vi "S1&S2_CHECK.vi"(8 "Message 2":string, 9 "MODE":string, 11 "task/channels in":refnum<k21>="CHECK_STS_S1") -> (3 "S1Bit_out":string)   [LabVIEW 2011]
uses:
  <vilib>/DAQmx/read.llb/DAQmx Read (Digital 1D Bool 1Chan 1Samp).vi
panel:
  out "Message":string
  out "Time out":dbl(slide) scale=0.0..40.0
  out "DIP SWITCH":bool[](array[boolean])
  # "1"
  # "2"
  # "3"
  # "4"
  # "5"
  # "6"
  # "7"
  # "8"
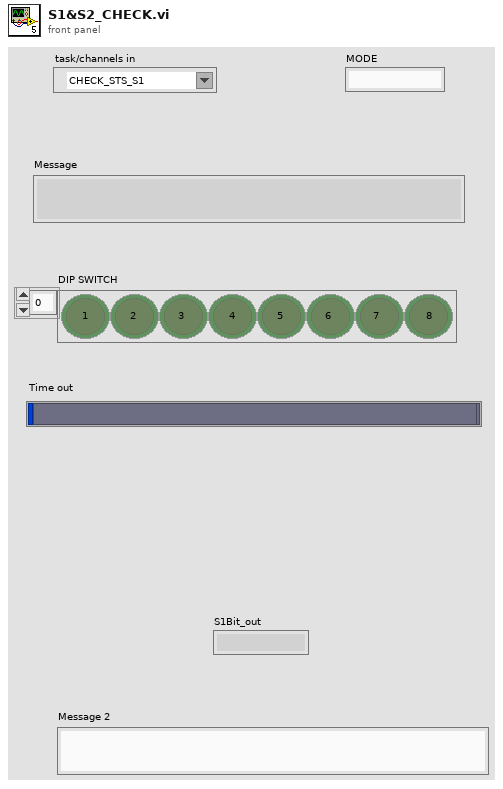
[diagram p1: front panel]
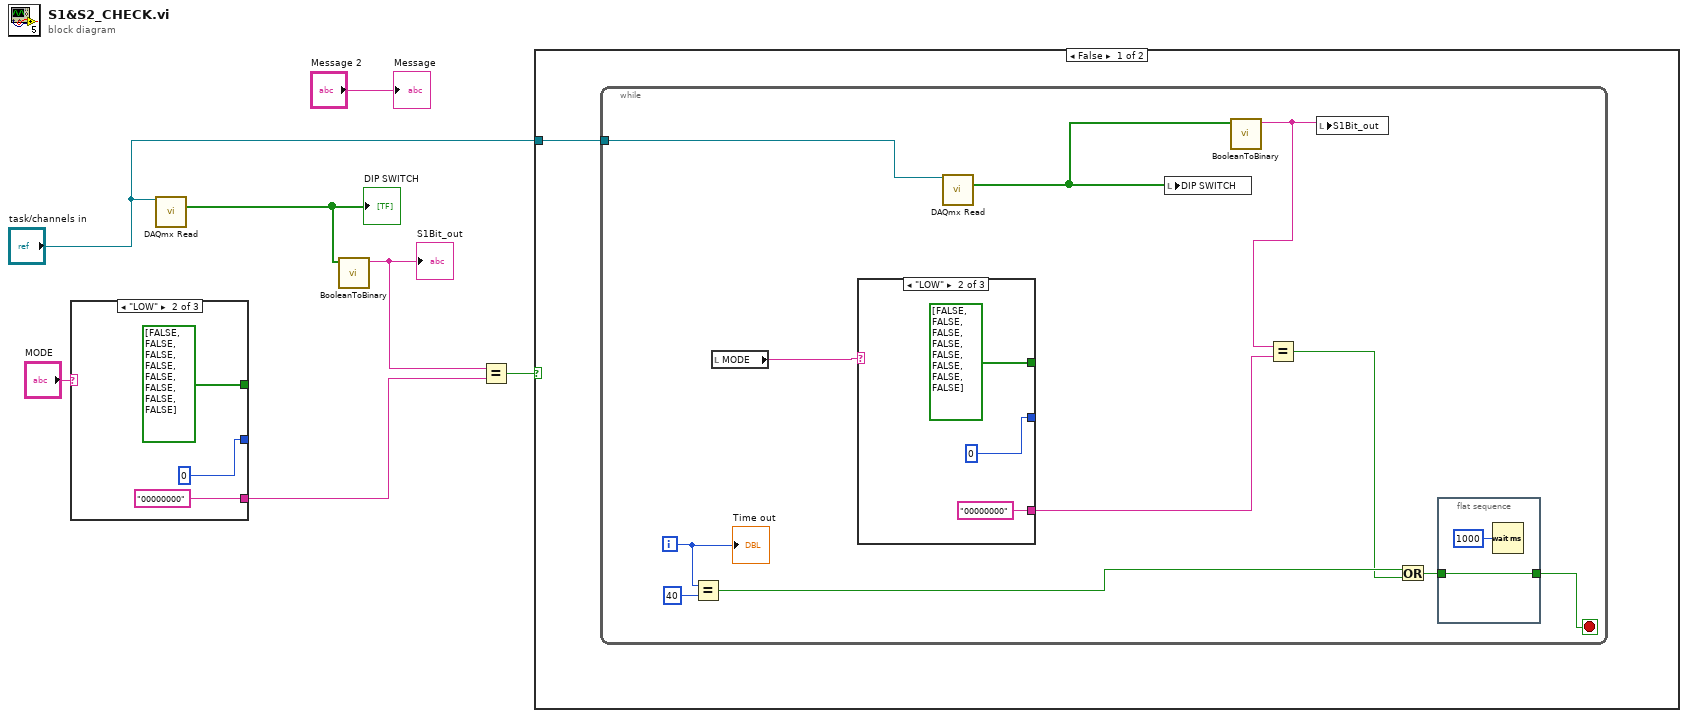
[diagram p0: block diagram]
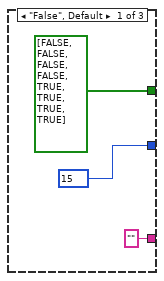
[diagram p2: hidden frame]
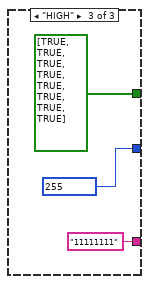
[diagram p3: hidden frame]
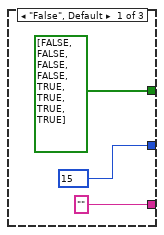
[diagram p5: hidden frame]
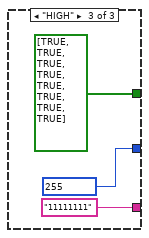
[diagram p6: hidden frame]
diagram:
  n1 = case shown="\"LOW\"" "MODE" {
    tunnel: [bool[] [FALSE, FALSE, FALSE, FALSE, TRUE, TRUE, TRUE, TRUE] ("y") bool[] [FALSE, FALSE, FALSE, FALSE, FALSE, FALSE, FALSE, FALSE] ("y") bool[] [TRUE, TRUE, TRUE, TRUE, TRUE, TRUE, TRUE, TRUE] ("y")] -> _
    tunnel: [u32 15 ("FF") u32 0 ("FF") u32 255 ("FF")] -> _
    tunnel: ["" "00000000" "11111111"] -> w1
    frame "False", Default {
    }
    frame "LOW" {
    }
    frame "HIGH" {
    }
  }
  n2 = call-poly <vilib>:"DAQmx Read.vi"("task/channels in"="task/channels in") -> ("data"=w3:bool[])  [unwired: 12 in, 2 out]
  "DIP SWITCH" <- w3
  n3 = call "BooleanToBinary.vi"("data"=w3) -> ("BinaryOut"=w2:string)  [unwired: 10 in]
  "S1Bit_out" <- w2
  n4 = Equal?(x=w2, y=w1) -> (x = y?=w7:bool)
  n5 = case shown="False" w7 {
    tunnel: "task/channels in" -> [w17 _]
    frame False {
      n6 = while {
        tunnel: w17 -> [w21]
        i -> [w28]
        stop <- w23 stop-if-true
        n7 = Equal?(x=w28, y=40) -> (x = y?=w26:bool)
        n8 = local read "MODE"() -> (w25:string)
        n9 = case shown="\"LOW\"" w25 {
          tunnel: [bool[] [FALSE, FALSE, FALSE, FALSE, TRUE, TRUE, TRUE, TRUE] ("y") bool[] [FALSE, FALSE, FALSE, FALSE, FALSE, FALSE, FALSE, FALSE] ("y") bool[] [TRUE, TRUE, TRUE, TRUE, TRUE, TRUE, TRUE, TRUE] ("y")] -> _
          tunnel: [u32 15 ("FF") u32 0 ("FF") u32 255 ("FF")] -> _
          tunnel: ["" "00000000" "11111111"] -> w18
          frame "False", Default {
          }
          frame "LOW" {
          }
          frame "HIGH" {
          }
        }
        n10 = call-poly <vilib>:"DAQmx Read.vi"("task/channels in"=w21) -> ("data"=w20:bool[])  [unwired: 12 in, 2 out]
        n11 = local write "DIP SWITCH"(w20) -> ()
        n12 = call "BooleanToBinary.vi"("data"=w20) -> ("BinaryOut"=w19:string)  [unwired: 10 in]
        n13 = Equal?(x=w19, y=w18) -> (x = y?=w24:bool)
        n14 = local write "S1Bit_out"(w19) -> ()
        n15 = Or(x=w26, y=w24) -> (x .or. y?=w22:bool)
        n16 = flat-sequence {
          tunnel: [w30] -> w23
          tunnel: w22 -> [w30]
          frame #0 {
            n17 = Wait (ms)(milliseconds to wait=u32 1000) -> ()  [unwired: 1 out]
          }
        }
        "Time out" <- w28
      }
    }
    frame True {
    }
  }
  "Message" <- "Message 2"
